vi "ToRepo.vi"(8 "error in":errorcluster, 9 "to repo cluster":T1, 10 "repository in":refnum<class "NISE_CEF_Repository.lvclass">, 11 "node in":refnum<class "CustomDevice.lvclass">) -> (0 "error out":errorcluster, 2 "repository out":refnum<class "NISE_CEF_Repository.lvclass">, 3 "node out":refnum<class "CustomDevice.lvclass">)   [LabVIEW 2019, in "CustomDevice.lvclass"]
doc: "Transfers the information from the tree node into the repo. How it is stored in the repo depends on the Repo.Copyright 2015 National Instruments Corporation\n\nLicensed under the Apache License, Version 2.0 (the \"License\"); you may not use this file except in compliance with the License. You may obtain a copy of the License at http://www.apache.org/licenses/LICENSE-2.0\nUnless required by applicable law or agreed to in writing, software distributed under the License is distributed on an \"AS IS\" BASIS, WITHOUT WARRANTIES OR CONDITIONS OF ANY KIND, either express or implied. See the License for the specific language governing permissions and limitations under the License."
uses:
  CustomDevice.lvclass
  <vilib>/NI/Configuration Framework/Repository/NISE_CEF_Repository.lvclass
  <vilib>/NI/Configuration Framework/Node/ToRepoCluster.ctl
  CustomDeviceRepo/CustomDeviceRepo.lvclass
  C:/Program Files (x86)/National Instruments/LabVIEW 2019/vi.lib/NI/Configuration Framework/Repository/NISE_CEF_Repository.lvclass
  CustomDevice.lvclass/CustomDevice.ctl
  CustomDeviceRepo/CustomDeviceRepo.lvclass/CustomDeviceRepo.ctl
  CustomDeviceRepo/Write Main CD Properties.vi
  <vilib>/NI/Configuration Framework/Node/NISE_CEF_Node.lvclass
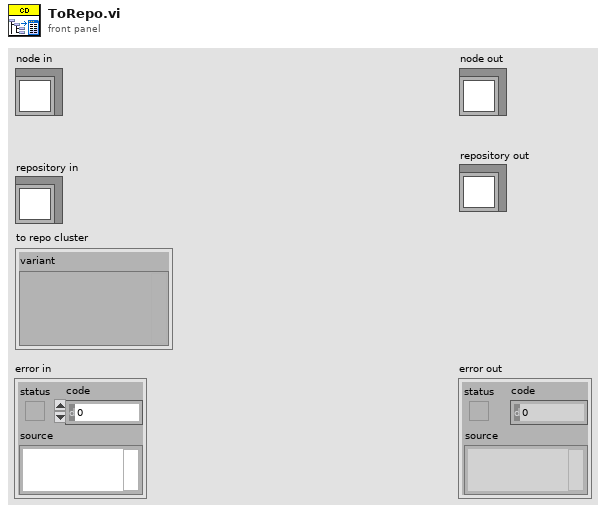
[diagram p1: front panel]
types:
  T1 = typedef "NISE_CEF_Node.lvclass/ToRepoCluster.ctl" = cluster{"variant":variant}
  T2 = typedef "VeriStand Custom Device XML Parser.lvlib/Main Custom Device Properties.ctl" = cluster{"CD Name":string, "Version":string, "Max Occurrences":i32, "Device Type":enum16{"Asynchronous", "Inline HW Interface", "Inline Model Interface", "Inline Timing and Sync", "Asynchronous Timing and Sync"}, "Main Page GUID":string}
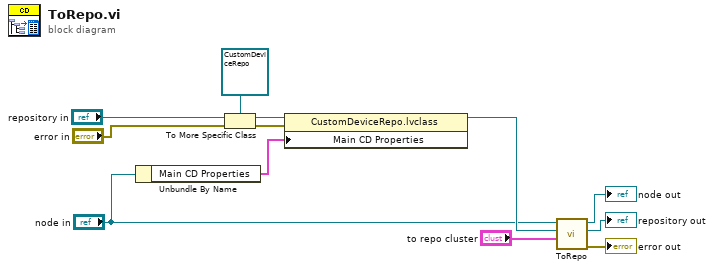
[diagram p0: block diagram]
diagram:
  n1 = Unbundle By Name("node in") -> ("Main CD Properties"=w3:T2)
  n2 = To More Specific Class(target class=refnum<class "CustomDeviceRepo.lvclass"> refnum ("CustomDeviceRepo.lvclass"), reference="repository in", error in="error in") -> (specific class reference=w5:refnum<class "CustomDeviceRepo.lvclass">, error out=w4:errorcluster)
  n3 = property class="CustomDeviceRepo.lvclass"(reference=w5, error in=w4, "Main CD Properties"=w3) -> (reference out=w2:refnum<class "CustomDeviceRepo.lvclass">)  [unwired: 1 out]
  n4 = call-parent "ToRepo.vi"("to repo cluster"="to repo cluster", "repository in"=w2, "node in"="node in") -> ("error out"=→"error out":errorcluster, "repository out"=→"repository out":refnum<class "NISE_CEF_Repository.lvclass">, "node out"=→"node out":refnum<class "CustomDevice.lvclass">)  [unwired: 6 in]
